vi "FixQueryString.vi"(4 "write buffer":string) -> (1 "write buffer fixed":string)   [LabVIEW 2015]
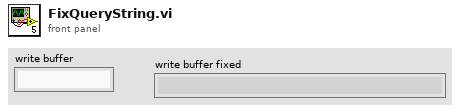
[diagram p1: front panel]
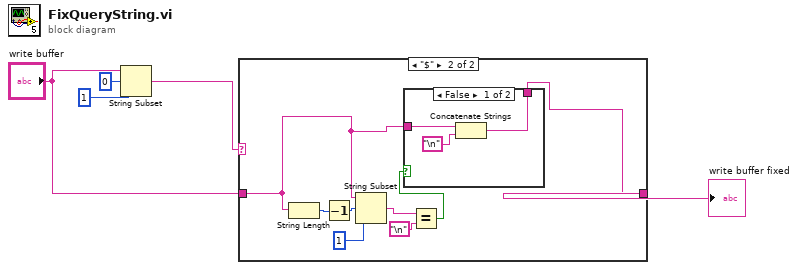
[diagram p0: block diagram]
diagram:
  n1 = String Subset(string="write buffer", offset (0)=0, length (rest)=1 ("length (rest)")) -> (substring=w3:string)
  n2 = case shown="\"$\"" w3 {
    tunnel: "write buffer" -> [w6 w8]
    tunnel: [w6 w7] -> w1
    frame "~", Default {
    }
    frame "$" {
      n3 = String Length(string=w8) -> (length=w14:i32)
      n4 = Decrement(x=w14) -> (x-1=w13:i32)
      n5 = String Subset(string=w8, offset (0)=w13, length (rest)=1 ("length (rest)")) -> (substring=w11:string)
      n6 = Equal?(x=w11, y="\n") -> (x = y?=w9:bool)
      n7 = case shown="False" w9 {
        tunnel: w8 -> [w17 w18]
        tunnel: [w15 w18] -> w7
        frame False {
          n8 = Concatenate Strings(w17, "\n") -> (w15:string)
        }
        frame True {
        }
      }
    }
  }
  "write buffer fixed" <- w1
